vi "Read Lead Res.vi"(8 "error in (no error)":errorcluster, 11 "Strain in":refnum<class "Strain.lvclass">) -> (0 "error out":errorcluster, 2 "Lead Res":dbl, 3 "Strain out":refnum<class "Strain.lvclass">)   [LabVIEW 2018, in "Measurement Channels.lvlib" / "Strain.lvclass"]
uses:
  Strain.lvclass
  Strain.lvclass/Strain.ctl
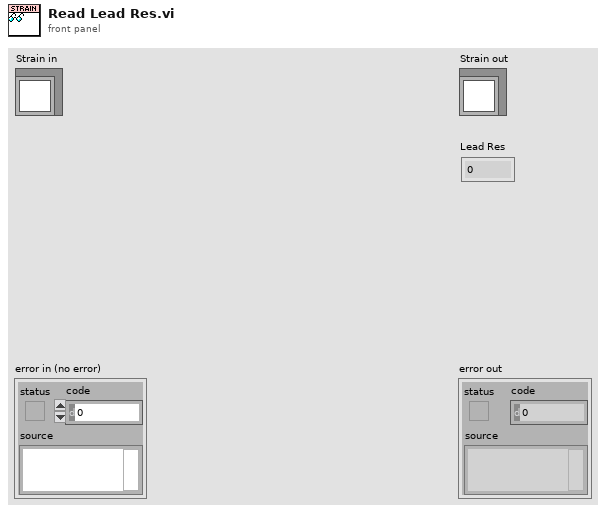
[diagram p1: front panel]
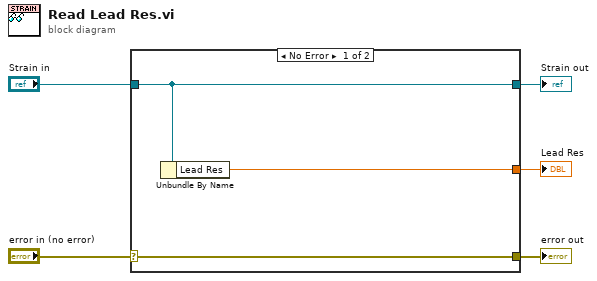
[diagram p0: block diagram]
diagram:
  n1 = case shown="No Error" "error in (no error)" {
    selector: "error in (no error)" -> [w8 w9]
    tunnel: [w8 w9] -> w4
    tunnel: [w7 w10] -> w2
    tunnel: "Strain in" -> [w7 w10]
    tunnel: [w6 _] -> w1
    frame No Error {
      n2 = Unbundle By Name(w7) -> ("Lead Res"=w6:dbl)
    }
    frame Error {
    }
  }
  "error out" <- w4
  "Strain out" <- w2
  "Lead Res" <- w1
